vi "FindCompDevItemID.vi"(8 "error in":errorcluster, 11 "VIProjectItem":refnum<vi>) -> (0 "error out":errorcluster, 2 "CompDevProjectItem":refnum<vi>, 3 "VIProjectItem":refnum<vi>)   [LabVIEW 2020, in "NI_Variable.lvlib"]
uses:
  <vilib>/variable/NI_Variable.lvlib
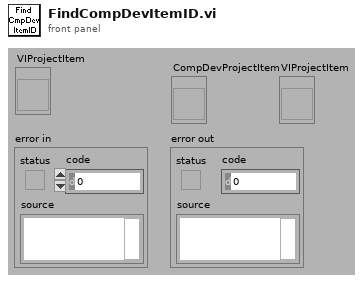
[diagram p1: front panel]
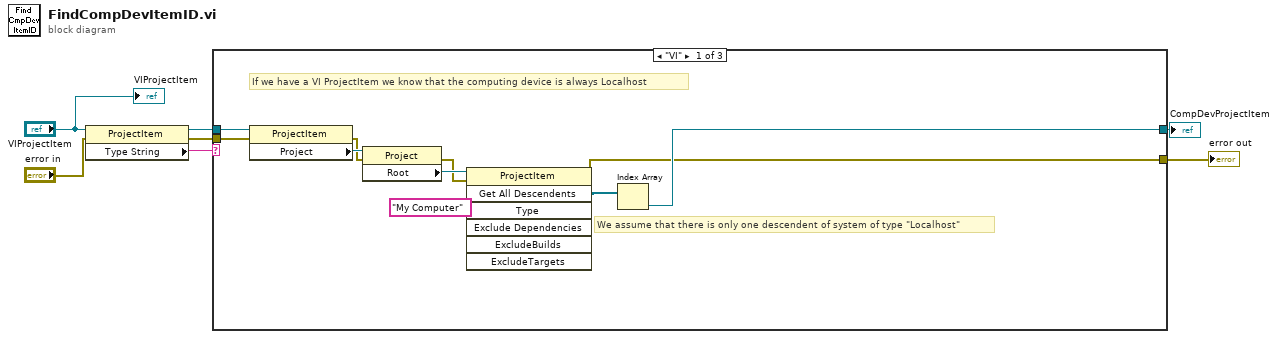
[diagram p0: block diagram]
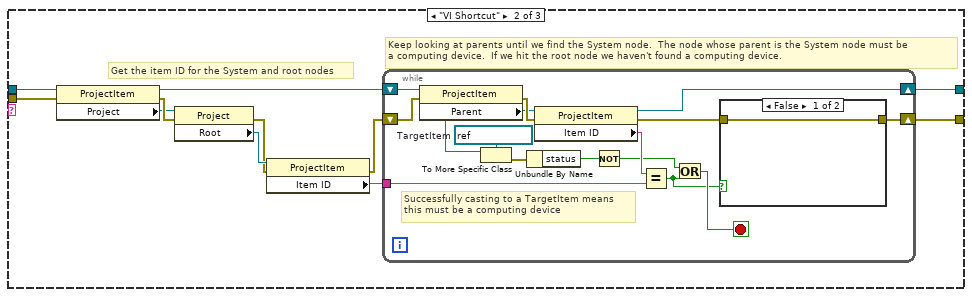
[diagram p2: hidden frame]
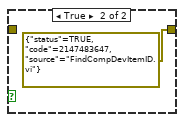
[diagram p3: hidden frame]
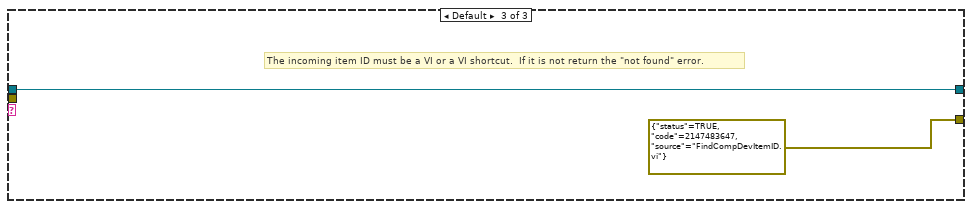
[diagram p4: hidden frame]
diagram:
  n1 = property class="ProjectItem"(reference="VIProjectItem", error in="error in") -> (reference out=w5:refnum<vi>, error out=w2:errorcluster, "Type String"=w4:string)
  n2 = case shown="\"VI\"" w4 {
    tunnel: w5 -> [w17 w28 w47]
    tunnel: [w9 w26 w47] -> w7
    tunnel: [w8 w24 errorcluster {"status"=TRUE, "code"=2147483647, "source"="FindCompDevItemID.vi"} ("error out")] -> w6
    tunnel: w2 -> [w15 w23 _]
    frame "VI" {
      # "We assume that there is only one descendent of system of type \"Localhost\""
      # "If we have a VI ProjectItem we know that the computing device is always Localhost"
      n3 = property class="ProjectItem"(reference=w17, error in=w15) -> (error out=w14:errorcluster, "Project"=w16:refnum<vi>)  [unwired: 1 out]
      n4 = property class="Project"(reference=w16, error in=w14) -> (error out=w11:errorcluster, "Root"=w12:refnum<vi>)  [unwired: 1 out]
      n5 = invoke class="ProjectItem" method="Get All Descendents"(reference=w12, error in=w11, "Type"="My Computer") -> (error out=w8:errorcluster, "All Descendents"=w10:refnum<vi>[])  [unwired: 4 in, 5 out]
      n6 = Index Array(array=w10) -> (element=w9:refnum<vi>)  [unwired: 1 in]
    }
    frame "VI Shortcut" {
      # "Keep looking at parents until we find the System node.  The node whose parent is the System node must be \na computing device.  If we hit the root node we haven't found a computing device."
      # "Get the item ID for the System and root nodes"
      n7 = property class="ProjectItem"(reference=w28, error in=w23) -> (reference out=w27:refnum<vi>, error out=w25:errorcluster, "Project"=w21:refnum<vi>)
      n8 = property class="Project"(reference=w21, error in=w25) -> (error out=w19:errorcluster, "Root"=w20:refnum<vi>)  [unwired: 1 out]
      n9 = property class="ProjectItem"(reference=w20, error in=w19) -> (error out=w18:errorcluster, "Item ID"=w22:string)  [unwired: 1 out]
      n10 = while {
        shift-right: [w35] -> w24
        shift-left: w18 -> [w42]
        shift-right: [w40] -> w26
        shift-left: w27 -> [w43]
        tunnel: w22 -> [w37]
        stop <- w39 stop-if-true
        w32 = refnum<vi> refnum  # TargetItem
        # "Successfully casting to a TargetItem means \nthis must be a computing device"
        n11 = property class="ProjectItem"(reference=w43, error in=w42) -> (error out=w41:errorcluster, "Parent"=w33:refnum<vi>)  [unwired: 1 out]
        n12 = To More Specific Class(target class=w32, reference=w33) -> (error out=w31:errorcluster)  [unwired: 1 in, 1 out]
        n13 = Unbundle By Name(w31) -> ("status"=w30:bool)
        n14 = property class="ProjectItem"(reference=w33, error in=w41) -> (reference out=w40:refnum<vi>, error out=w36:errorcluster, "Item ID"=w38:string)
        n15 = Not(x=w30) -> (.not. x?=w29:bool)
        n16 = Equal?(x=w38, y=w37) -> (x = y?=w34:bool)
        n17 = Or(x=w29, y=w34) -> (x .or. y?=w39:bool)
        n18 = case shown="False" w34 {
          tunnel: w36 -> [w44 _]
          tunnel: [w44 errorcluster {"status"=TRUE, "code"=2147483647, "source"="FindCompDevItemID.vi"} ("error out")] -> w35
          frame False {
          }
          frame True {
          }
        }
      }
    }
    frame Default {
      # "The incoming item ID must be a VI or a VI shortcut.  If it is not return the \"not found\" error."
    }
  }
  "CompDevProjectItem" <- w7
  "error out" <- w6
  "VIProjectItem" <- "VIProjectItem"
